vi "Update Online List.vi"(8 "error in (no error)":errorcluster, 10 "Online List":string[](array[string]), 11 "Chat Window Controller UI in":refnum<class "Chat Window Controller UI.lvclass">) -> (0 "error out":errorcluster, 3 "Chat Window Controller UI out":refnum<class "Chat Window Controller UI.lvclass">)   [LabVIEW 2020, in "Chat Window UI.lvlib" / "Chat Window Controller UI.lvclass"]
uses:
  Chat Window Controller UI.lvclass
  Chat Window Controller UI.lvclass/Chat Window Controller UI.ctl
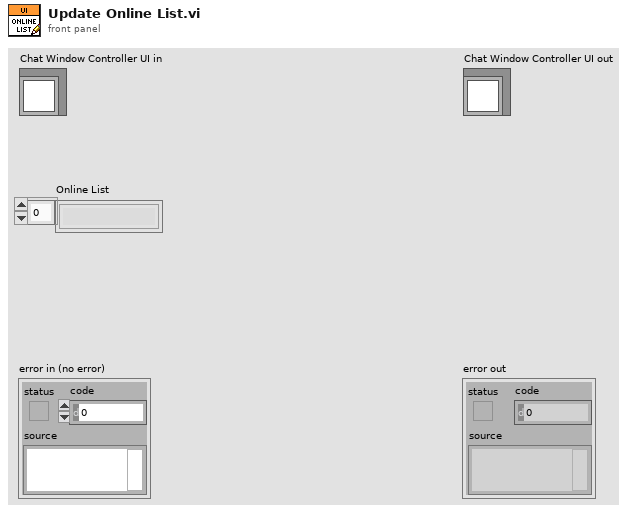
[diagram p1: front panel]
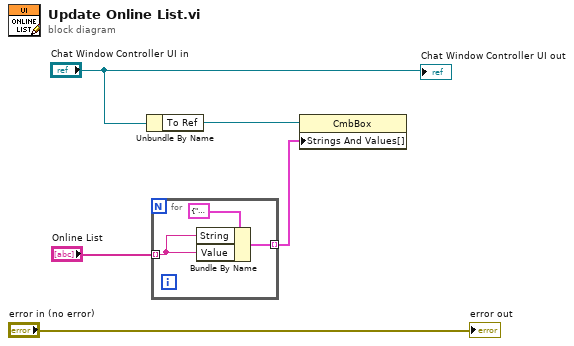
[diagram p0: block diagram]
diagram:
  n1 = Unbundle By Name("Chat Window Controller UI in") -> ("To Ref"=w3:refnum<vi>)
  n2 = for {
    tunnel: "Online List" -> [w7] mode=indexing
    tunnel: [w6] -> w1 mode=indexing
    n3 = Bundle By Name(cluster=cluster{"String":string, "Value":string} {"String"="", "Value"=""}, "String"=w7, "Value"=w7) -> (w6:cluster{"String":string, "Value":string})
  }
  n4 = property class="CmbBox"(reference=w3, "Strings And Values[]"=w1) -> ()  [unwired: 1 in, 2 out]
  "error out" <- "error in (no error)"
  "Chat Window Controller UI out" <- "Chat Window Controller UI in"
